vi "Select Next Path.vi"(0 "Auto Data":T1) -> (1 "Command Info":T3(array[cluster]), 3 "Current Limits":dbl, 4 "Velocities":T2[](array[typedef]), 6 "Positions":cluster{"x":dbl, "y":dbl, "th":dbl}[](array[cluster]), 8 "Number of Remaining Auto Paths":dbl, 10 "Zero Velocity?":bool[](array[boolean]), 14 "Auto Data Out":T1, 15 "Zero Translational Velocity?":bool[](array[boolean]))   [LabVIEW 2025]
uses:
  Implementation/Auto Data.ctl
  swerve-template/Type Definitions/Data/Robot Velocities.ctl
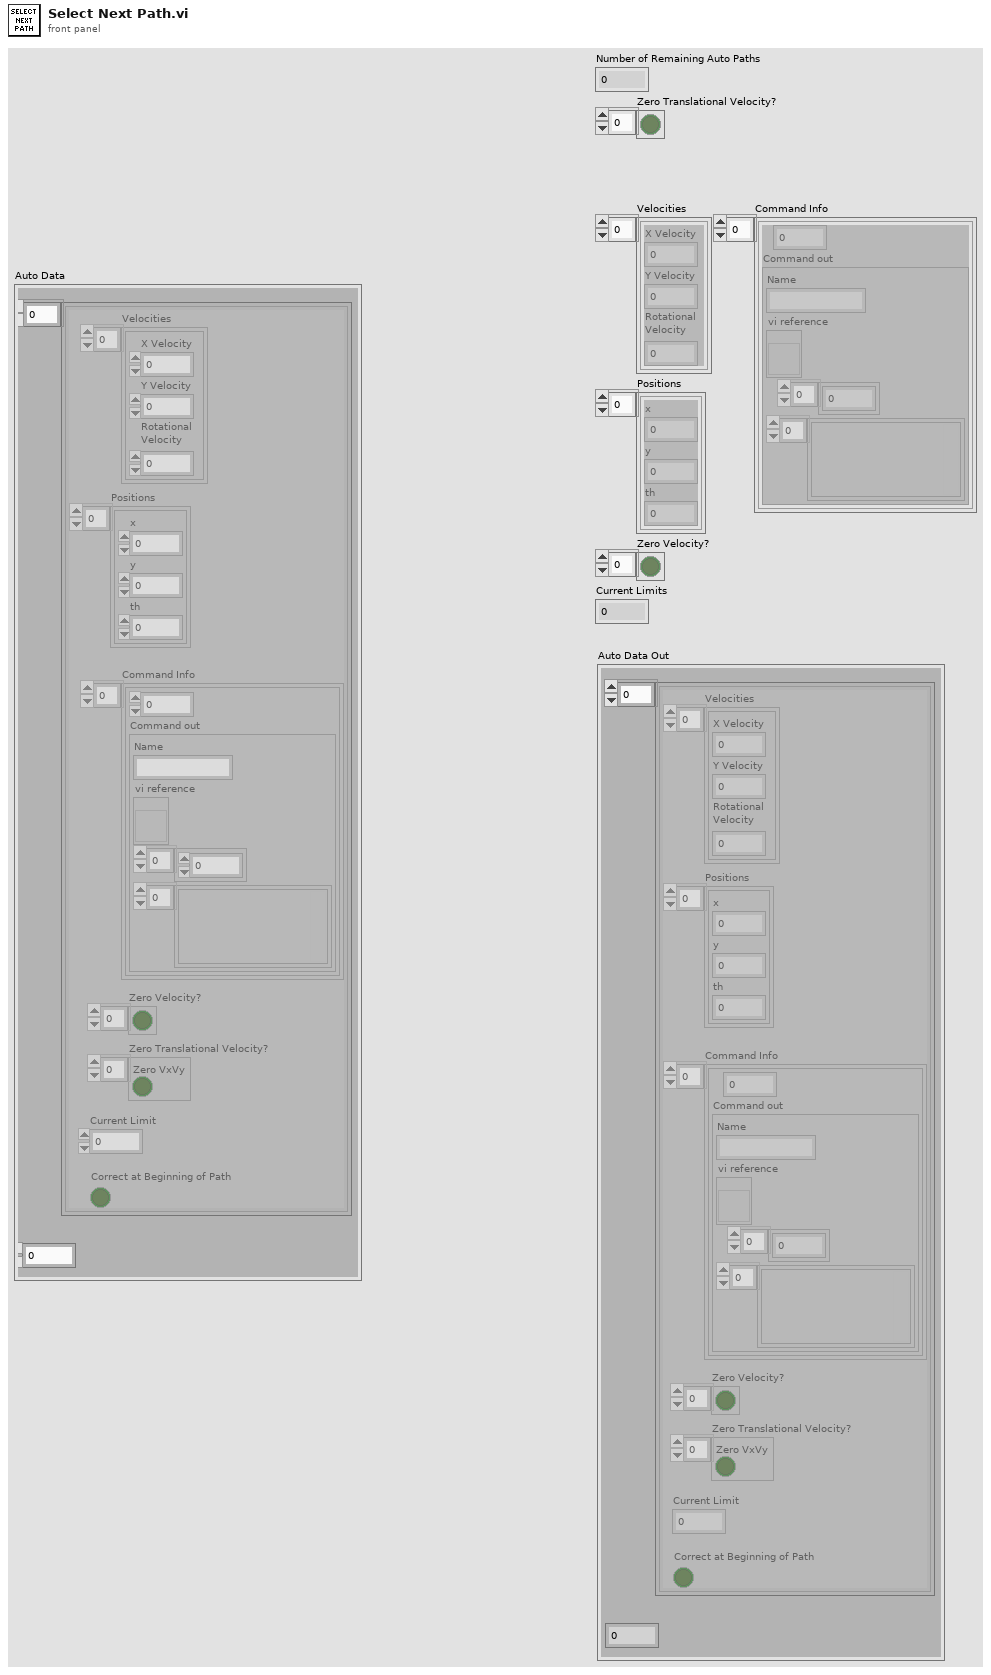
[diagram p1: front panel]
types:
  T1 = typedef "Auto Data.ctl" = cluster{"Auto Data":cluster{"Velocities":T2[], "Positions":cluster{"x":dbl, "y":dbl, "th":dbl}[], "Command Info":cluster{dbl, "Command out":cluster{"Name":string, "vi reference":refnum<vi>, i32[], variant[]}}[], "Zero Velocity?":bool[], "Zero Translational Velocity?":bool[], "Current Limit":dbl, "Correct at Beginning of Path":bool}[], "Number of Remaining Auto Paths":dbl}
  T2 = typedef "Robot Velocities.ctl" = cluster{"X Velocity":dbl, "Y Velocity":dbl, "Rotational \nVelocity":dbl}
  T3 = cluster{dbl, "Command out":cluster{"Name":string, "vi reference":refnum<vi>, i32[], variant[]}}[]
  T4 = cluster{"Velocities":T2[], "Positions":cluster{"x":dbl, "y":dbl, "th":dbl}[], "Command Info":cluster{dbl, "Command out":cluster{"Name":string, "vi reference":refnum<vi>, i32[], variant[]}}[], "Zero Velocity?":bool[], "Zero Translational Velocity?":bool[], "Current Limit":dbl, "Correct at Beginning of Path":bool}[]
  T5 = cluster{"Velocities":T2[], "Positions":cluster{"x":dbl, "y":dbl, "th":dbl}[], "Command Info":cluster{dbl, "Command out":cluster{"Name":string, "vi reference":refnum<vi>, i32[], variant[]}}[], "Zero Velocity?":bool[], "Zero Translational Velocity?":bool[], "Current Limit":dbl, "Correct at Beginning of Path":bool}
  T6 = cluster{cluster{"Velocities":T2[], "Positions":cluster{"x":dbl, "y":dbl, "th":dbl}[], "Command Info":cluster{dbl, "Command out":cluster{"Name":string, "vi reference":refnum<vi>, i32[], variant[]}}[], "Zero Velocity?":bool[], "Zero Translational Velocity?":bool[], "Current Limit":dbl, "Correct at Beginning of Path":bool}[], dbl}
  T7 = cluster{"Auto Data":cluster{"Velocities":T2[], "Positions":cluster{"x":dbl, "y":dbl, "th":dbl}[], "Command Info":cluster{dbl, "Command out":cluster{"Name":string, "vi reference":refnum<vi>, i32[], variant[]}}[], "Zero Velocity?":bool[], "Zero Translational Velocity?":bool[], "Current Limit":dbl, "Correct at Beginning of Path":bool}[], "Number of Remaining Auto Paths":dbl}
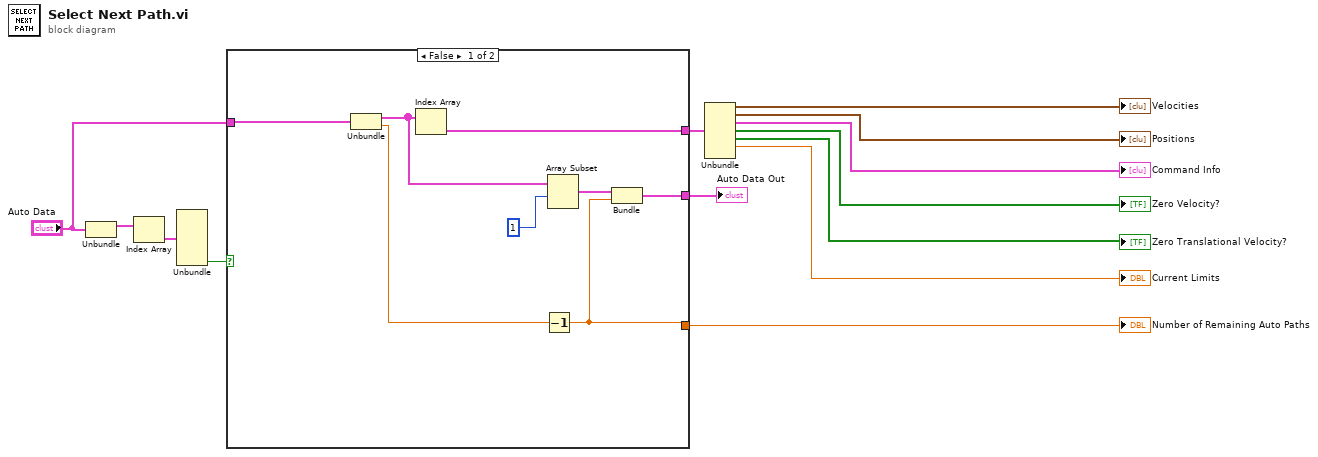
[diagram p0: block diagram]
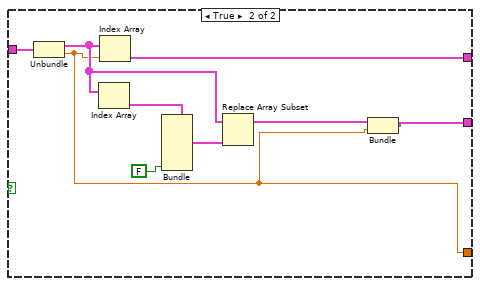
[diagram p2: hidden frame]
diagram:
  n1 = Unbundle("Auto Data") -> ("Auto Data"=w11:T4)  [unwired: 1 out]
  n2 = Index Array(array=w11) -> (element=w10:T5)  [unwired: 1 in]
  n3 = Unbundle(w10) -> ("Correct at Beginning of Path"=w9:bool)  [unwired: 6 out]
  n4 = case shown="False" w9 {
    tunnel: "Auto Data" -> [w21 w30]
    tunnel: [w20 w29] -> w13
    tunnel: [w17 w22] -> w8
    tunnel: [w15 w23] -> w1
    frame False {
      n5 = Unbundle(w21) -> ("Auto Data"=w18:T4, "Number of Remaining Auto Paths"=w19:dbl)
      n6 = Index Array(array=w18) -> (element=w20:T5)  [unwired: 1 in]
      n7 = Decrement(x=w19) -> (x-1=w17:dbl)
      n8 = Array Subset(array=w18, index=1) -> (w16:T4)  [unwired: 1 in]
      n9 = Bundle(w16, w17) -> (w15:T6)  [unwired: 1 in]
    }
    frame True {
      n10 = Unbundle(w30) -> ("Auto Data"=w25:T4, "Number of Remaining Auto Paths"=w22:dbl)
      n11 = Index Array(array=w25) -> (element=w28:T5)  [unwired: 1 in]
      n12 = Index Array(array=w25, index=w22) -> (element=w29:T5)
      n13 = Bundle(cluster=w28, "Correct at Beginning of Path"=FALSE) -> (w26:T5)  [unwired: 6 in]
      n14 = Replace Array Subset(array=w25, new element=w26) -> (w24:T4)  [unwired: 1 in]
      n15 = Bundle("Auto Data"=w24, "Number of Remaining Auto Paths"=w22) -> (w23:T7)  [unwired: 1 in]
    }
  }
  "Number of Remaining Auto Paths" <- w8
  "Auto Data Out" <- w1
  n16 = Unbundle(w13) -> ("Velocities"=→"Velocities":T2[], "Positions"=→"Positions":cluster{"x":dbl, "y":dbl, "th":dbl}[], "Command Info"=→"Command Info":T3, "Zero Velocity?"=→"Zero Velocity?":bool[], "Zero Translational Velocity?"=→"Zero Translational Velocity?":bool[], "Current Limit"=→"Current Limits":dbl)  [unwired: 1 out]
